vi "init.vi"(8 "error in (no error)":errorcluster, 10 "Resource":string, 11 "FgenNiPxi in":refnum<class "ArbNi.lvclass">) -> (0 "error out":errorcluster, 3 "FgenNiPxi out":refnum<class "ArbNi.lvclass">)   [LabVIEW 2023, in "ArbNi.lvclass"]
doc: "<b>Author:</b> Wolfgang\n<b>Description:</b> Method to initialize an instrument by resource name (defined in NI MAX) for any instrument category."
uses:
  ArbNi.lvclass
  <instrlib>/niFgen/niFgen.llb/niFgen Output Mode.ctl
  <instrlib>/niFgen/niFgen.llb/niFgen Output Impedance.ctl
  ArbNi.lvclass/ArbNi.ctl
  Arb.lvclass
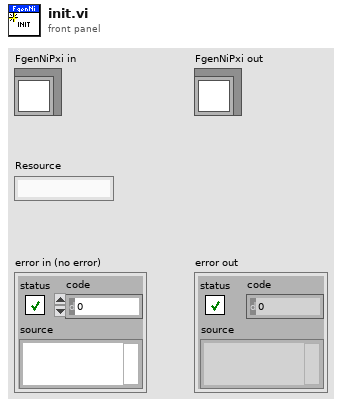
[diagram p1: front panel]
types:
  T1 = typedef "niFgen Output Impedance.ctl" = i32
  T2 = typedef "niFgen Output Mode.ctl" = u32
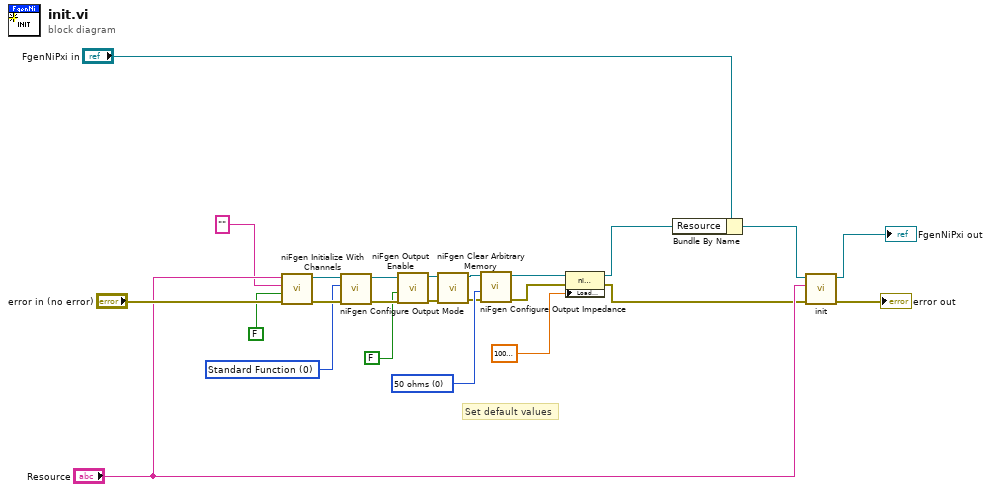
[diagram p0: block diagram]
diagram:
  w10 = T1 0 items=["50 ohms", "75 ohms"] ("Impedance (default: 0=50 ohms)")
  w15 = T2 0 items=["Standard Function", "Frequency List", "Arbitrary Waveform", "Arbitrary Sequence", "Script"] ("Output Mode (default: 0=Standard Function)")
  # "Set default values"
  n1 = call <instrlib>:"niFgen Initialize With Channels.vi"("error in (no error)"="error in (no error)", "Reset Device (default: True)"=FALSE, "Channel Name"="", "Resource Name"="Resource") -> ("error out"=w16:errorcluster, "Instrument Handle Out"=w17:refnum<k15>)  [unwired: 6 in]
  n2 = call <instrlib>:"niFgen Configure Output Mode.vi"("error in (no error)"=w16, "Output Mode (default: 0=Standard Function)"=w15, "Instrument Handle"=w17) -> ("error out"=w13:errorcluster, "Instrument Handle Out"=w14:refnum<k15>)  [unwired: 6 in]
  n3 = call <instrlib>:"niFgen Output Enable.vi"("error in (no error)"=w13, "Output Enable (default: True)"=FALSE, "Instrument Handle"=w14) -> ("error out"=w3:errorcluster, "Instrument Handle Out"=w6:refnum<k15>)  [unwired: 7 in]
  n4 = call <instrlib>:"niFgen Clear Arbitrary Memory.vi"("error in (no error)"=w3, "Instrument Handle"=w6) -> ("error out"=w4:errorcluster, "Instrument Handle Out"=w5:refnum<k15>)  [unwired: 8 in]
  n5 = call <instrlib>:"niFgen Configure Output Impedance.vi"("error in (no error)"=w4, "Impedance (default: 0=50 ohms)"=w10, "Instrument Handle"=w5) -> ("error out"=w7:errorcluster, "Instrument Handle Out"=w9:refnum<k15>)  [unwired: 7 in]
  n6 = property class="niFgen"(reference=w9, error in=w7, "Load Impedance"=10000000000.0 ("Output:Load Impedance")) -> (reference out=w1:refnum<k15>, error out=w19:errorcluster)
  n7 = Bundle By Name(cluster="FgenNiPxi in", "Resource"=w1) -> (w22:refnum<class "ArbNi.lvclass">)
  n8 = call-parent "init.vi"("error in (no error)"=w19, "Resource"="Resource", "Instrument in"=w22) -> ("error out"=→"error out":errorcluster, "Instrument out"=→"FgenNiPxi out":refnum<class "ArbNi.lvclass">)  [unwired: 7 in]
